vi "_PC_Pub_Display_SysMsg.vi"(8 "error in (no error)":errorcluster, 10 "Msg String":string, 11 "SysMsg Ref In":refnum<vi>) -> (0 "error out":errorcluster, 3 "SysMsg Ref Out":refnum<vi>)   [LabVIEW 2018]
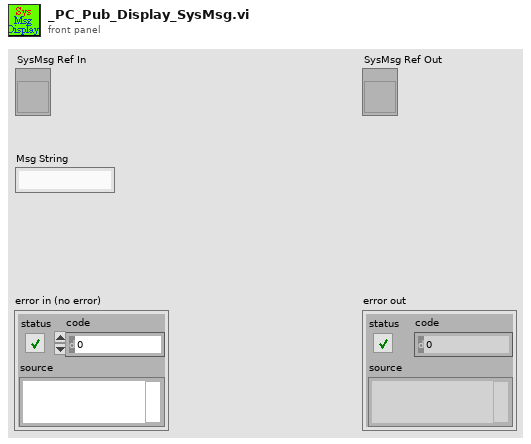
[diagram p1: front panel]
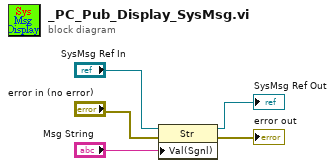
[diagram p0: block diagram]
diagram:
  n1 = property class="Str"(reference="SysMsg Ref In", error in="error in (no error)", "Val(Sgnl)"="Msg String") -> (reference out=→"SysMsg Ref Out":refnum<vi>, error out=→"error out":errorcluster)
